vi "Check Plugins.vi"(8 "error in (no error)":errorcluster, 11 "GUI Manager Module in":refnum<class "GUI Manager Module.lvclass">) -> (0 "error out":errorcluster, 3 "GUI Manager Module out":refnum<class "GUI Manager Module.lvclass">)   [LabVIEW 2020, in "VolatusGUI.lvlib" / "GUI Manager Module.lvclass"]
uses:
  GUI Manager Module.lvclass
  GUI Manager Module.lvclass/GUI Manager Module.ctl
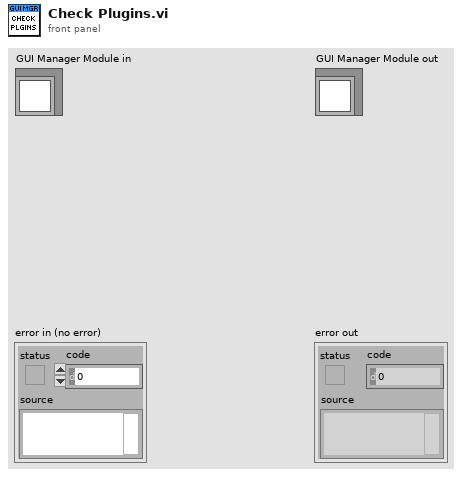
[diagram p1: front panel]
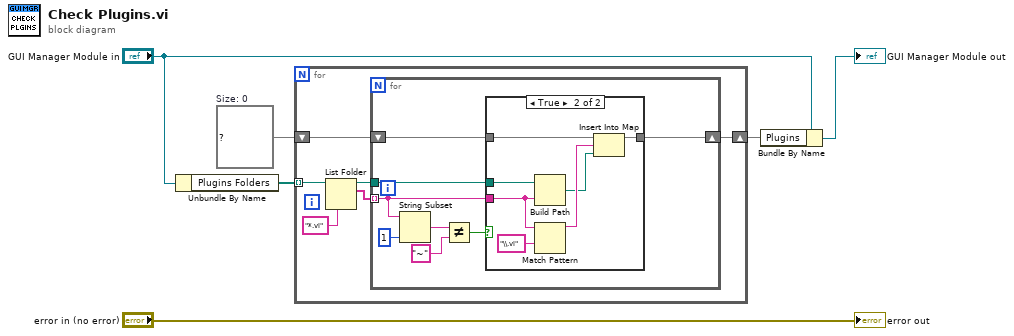
[diagram p0: block diagram]
diagram:
  w3 = map{string, path} {}  # Size: 0
  n1 = Unbundle By Name("GUI Manager Module in") -> ("Plugins Folders"=w4:path[])
  n2 = for {
    tunnel: w4 -> [w12] mode=indexing
    shift-right: [w7] -> w1
    shift-left: w3 -> [w8]
    n3 = List Folder(path=w12, pattern="*.vi") -> (path out=w9:path, filenames=w10:string[])  [unwired: 2 in, 2 out]
    n4 = for {
      tunnel: w10 -> [w17] mode=indexing
      tunnel: w9 -> [w20]
      shift-right: [w18] -> w7
      shift-left: w8 -> [w19]
      n5 = String Subset(string=w17, length (rest)=1 ("length (rest)")) -> (substring=w15:string)  [unwired: 1 in]
      n6 = Not Equal?(x=w15, y="~") -> (x != y?=w13:bool)
      n7 = case shown="True" w13 {
        tunnel: w20 -> [_ w28]
        tunnel: w19 -> [w21 w26]
        tunnel: [w21 w23] -> w18
        tunnel: w17 -> [_ w22]
        frame False {
        }
        frame True {
          n8 = Build Path(base path=w28, name or relative path=w22) -> (appended path=w24:path)
          n9 = Match Pattern(string=w22, regular expression="\\.vi") -> (before substring=w25:string)  [unwired: 1 in, 3 out]
          n10 = Insert Into Map(map in=w26, key=w25, value=w24) -> (map out=w23:map{string, path})  [unwired: 2 out]
        }
      }
    }
  }
  n11 = Bundle By Name(cluster="GUI Manager Module in", "Plugins"=w1) -> (→"GUI Manager Module out":refnum<class "GUI Manager Module.lvclass">)
  "error out" <- "error in (no error)"
